vi "Shutting Down.vi"(11 "Exit":T1) -> (3 "Quit?":bool)   [LabVIEW 2017]
uses:
  <extravilib>/ChannelInstances/Messenger-bool/))Channel.ctl
  <extravilib>/ChannelInstances/Messenger-bool/Read With Abort.vi
  <resource>/Channels/Messenger/Read With Abort.vi
  <vilib>/ChannelSupport/Channel Message/Read ID.vi
  <resource>/Channels/Messenger/Endpoint.vi
  <extravilib>/ChannelInstances/Messenger-bool/Unwrap.vi
  <extravilib>/ChannelInstances/Messenger-bool.lvlib
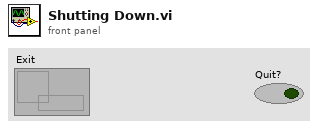
[diagram p1: front panel]
types:
  T1 = typedef "Messenger-bool.lvlib/))Channel.ctl" = refnum<queue>
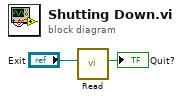
[diagram p0: block diagram]
diagram:
  n1 = call <extravilib>:"Read.vi"("channel"="Exit") -> ("element"=→"Quit?":bool)  [unwired: 7 in, 3 out]
